vi "Render.vi"(8 "error in (no error)":errorcluster, 10 "String in":string, 11 "OrderedList in":refnum<class "UnorderedList.lvclass">) -> (0 "error out":errorcluster, 2 "String out":string, 3 "OrderedList out":refnum<class "UnorderedList.lvclass">)   [LabVIEW 2021, in "LvMarkdown.lvlib" / "UnorderedList.lvclass"]
uses:
  UnorderedList.lvclass
  UnorderedList.lvclass/UnorderedList.ctl
  Collection/GetElements.vi
  IRenderable/IRenderable.lvclass
  Collection/Collection.lvclass
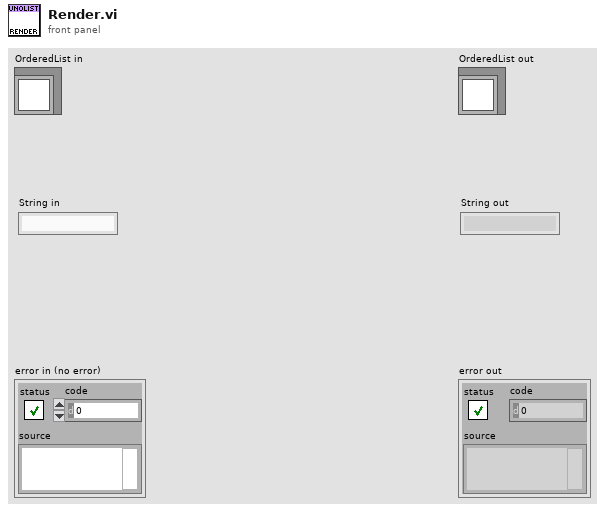
[diagram p1: front panel]
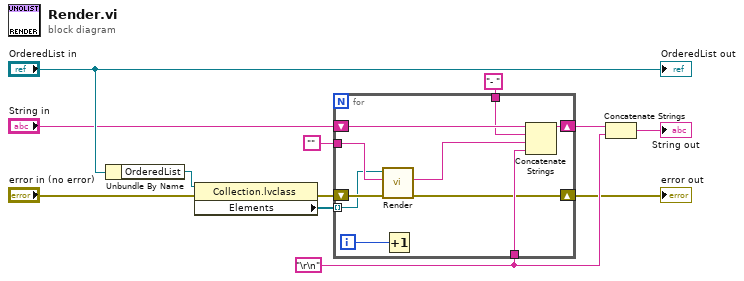
[diagram p0: block diagram]
diagram:
  w8 = "\r\n"
  n1 = Unbundle By Name("OrderedList in") -> ("OrderedList"=w11:refnum<class "Collection.lvclass">)
  n2 = property class="Collection.lvclass"(reference=w11, error in="error in (no error)") -> (error out=w2:errorcluster, "Elements"=w1:refnum<class "IRenderable.lvclass">[])  [unwired: 1 out]
  n3 = for {
    shift-right: [w21] -> w9
    shift-left: "String in" -> [w22]
    tunnel: w8 -> [w18]
    tunnel: "" -> [w16]
    shift-right: [w15] -> w5
    shift-left: w2 -> [w17]
    tunnel: "- " ("format string") -> [w13]
    tunnel: w1 -> [w14] mode=indexing
    i -> [w20]
    n4 = call-dynamic "Render.vi"("error in (no error)"=w17, "String in"=w16, "IRenderable in"=w14) -> ("error out"=w15:errorcluster, "String out"=w19:string)  [unwired: 6 in, 1 out]
    n5 = Increment(x=w20) -> ()  [unwired: 1 out]
    n6 = Concatenate Strings(w22, w13, w19, w18) -> (w21:string)
  }
  "error out" <- w5
  n7 = Concatenate Strings(w9, w8) -> (→"String out":string)
  "OrderedList out" <- "OrderedList in"
